vi "DefineFont.vi"(8 "error in (no error)":errorcluster) -> (0 "error out":errorcluster, 3 "Font out":refnum<class "Font.lvclass">)   [LabVIEW 2014, in "Font.lvclass"]
uses:
  Font.lvclass
  System.Drawing
  Font.lvclass/Font.ctl
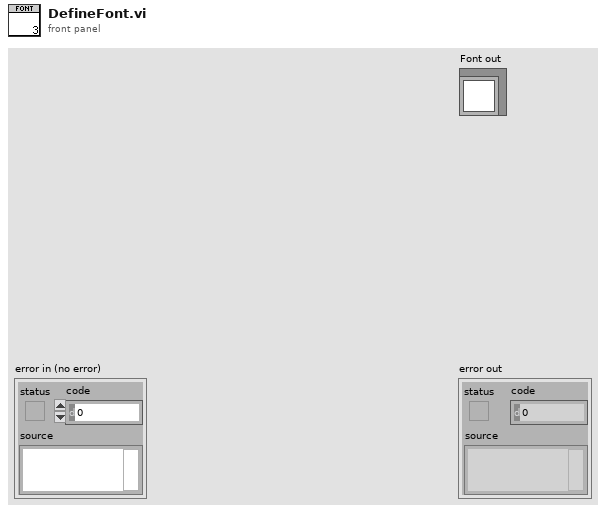
[diagram p1: front panel]
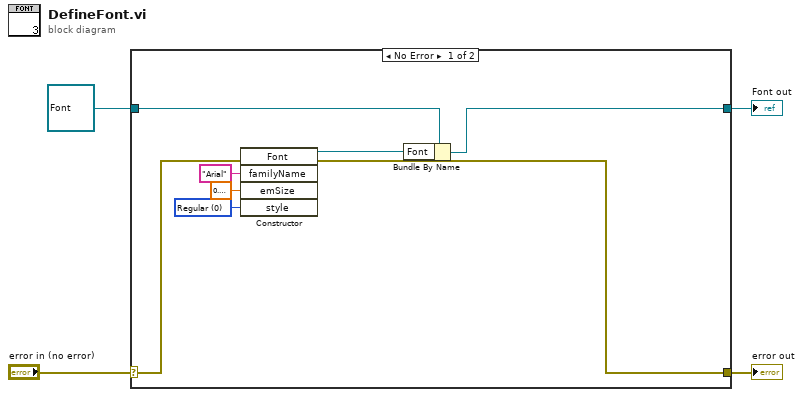
[diagram p0: block diagram]
diagram:
  n1 = case shown="No Error" "error in (no error)" {
    selector: "error in (no error)" -> [w8 w14]
    tunnel: [w5 w14] -> w3
    tunnel: [w6 w13] -> w1
    tunnel: refnum<class "Font.lvclass"> refnum ("Font in") -> [w7 w13]
    frame No Error {
      w11 = 0 items=["Regular"=0, "Bold"=1, "Italic"=2, "Underline"=4, "Strikeout"=8] ("style")
      n2 = constructor class="Font"(error in=w8, "familyName"="Arial", "emSize"=sgl 0.3, "style"=w11) -> (reference out=w9:refnum<k24>, error out=w5:errorcluster)  [unwired: 2 in, 4 out]
      n3 = Bundle By Name(cluster=w7, "Font"=w9) -> (w6:refnum<class "Font.lvclass">)
    }
    frame Error {
    }
  }
  "error out" <- w3
  "Font out" <- w1
